vi "語系切換.vi"(8 "error in":errorcluster, 9 "Control Array":refnum<vi>[](array[refnum]), 10 "Language":string, 11 "File Path Control":path) -> (0 "error out":errorcluster)   [LabVIEW 2015]
uses:
  <vilib>/Utility/config.llb/Read Key (String).vi
  <vilib>/Utility/config.llb/NI_LVConfig.lvlib
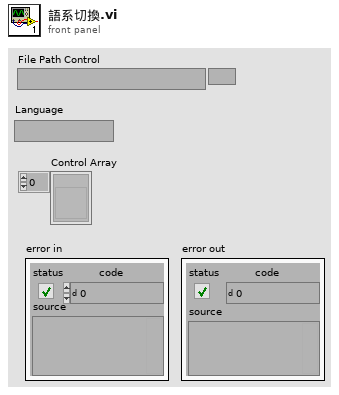
[diagram p1: front panel]
types:
  T1 = typedef "NI_LVConfig.lvlib/Config Data RefNum.ctl" = refnum<k1>
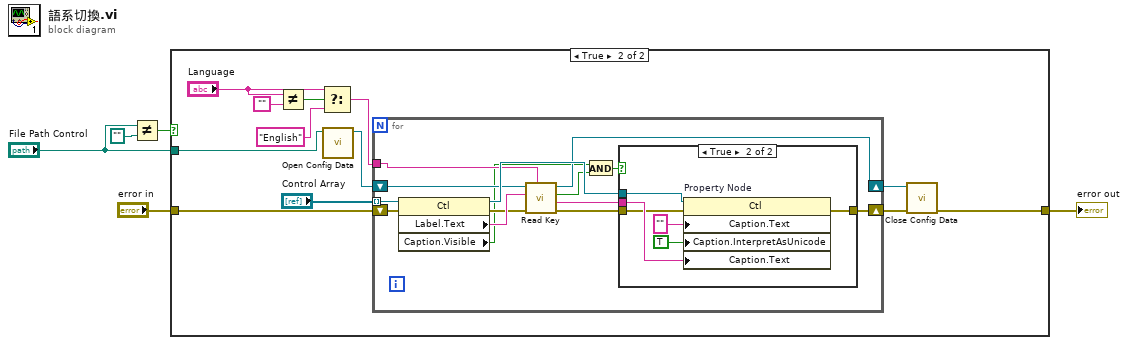
[diagram p0: block diagram]
diagram:
  n1 = Not Equal?(x="File Path Control", y=path "") -> (x != y?=w2:bool)
  n2 = case shown="True" w2 {
    tunnel: [w6 w8] -> w5
    tunnel: "File Path Control" -> [_ w15]
    tunnel: "error in" -> [w6 w10]
    frame False {
    }
    frame True {
      n3 = Not Equal?(x="Language", y="") -> (x != y?=w13:bool)
      n4 = Select(t="Language", s=w13, f="English") -> (s? t:f=w11:string)
      n5 = call <vilib>:"Open Config Data.vi"("configuration file path"=w15) -> ("refnum"=w18:T1)  [unwired: 8 in, 2 out]
      n6 = for {
        tunnel: "Control Array" -> [w28] mode=indexing
        tunnel: w11 -> [w31]
        shift-right: [w26] -> w16
        shift-left: w10 -> [w25]
        shift-right: [w22] -> w17
        shift-left: w18 -> [w23]
        n7 = property class="Ctl"(reference=w28, error in=w25) -> (reference out=w32:refnum<vi>, error out=w24:errorcluster, "Label.Text"=w29:string, "Caption.Visible"=w19:bool)
        n8 = call-poly <vilib>:"Read Key.vi"("section"=w31, "error in (no error)"=w24, "key"=w29, "refnum"=w23) -> ("error out"=w27:errorcluster, "value"=w30:string, "found?"=w21:bool, "refnum out"=w22:T1)  [unwired: 4 in]
        n9 = And(x=w19, y=w21) -> (x .and. y?=w20:bool)
        n10 = case shown="True" w20 {
          tunnel: w32 -> [_ w38]
          tunnel: w30 -> [_ w35]
          tunnel: w27 -> [w33 w34]
          tunnel: [w33 w39] -> w26
          frame False {
          }
          frame True {
            n11 = property on="Property Node" class="Ctl"(reference=w38, error in=w34, "Caption.Text"="", "Caption.InterpretAsUnicode"=TRUE ("Caption.Interpret As Unicode"), "Caption.Text"=w35) -> (error out=w39:errorcluster)  [unwired: 1 out]
          }
        }
      }
      n12 = call <vilib>:"Close Config Data.vi"("error in (no error)"=w16, "refnum"=w17) -> ("error out"=w8:errorcluster)  [unwired: 8 in, 1 out]
    }
  }
  "error out" <- w5
